vi "SendCommandTo8742.vi"(8 "error in (no error)":errorcluster, 10 "Command":string, 11 "PicoMotor8742Comm in":refnum<class "PicoMotor8742Comm.lvclass">) -> (0 "error out":errorcluster, 2 "Reply":string, 3 "PicoMotor8742Comm out":refnum<class "PicoMotor8742Comm.lvclass">)   [LabVIEW 2020, in "PicoMotor8742Comm.lvclass"]
uses:
  PicoMotor8742Comm.lvclass
  PicoMotor8742Comm.lvclass/PicoMotor8742Comm.ctl
  ASCIICommClass/ASCIICommClass.lvclass
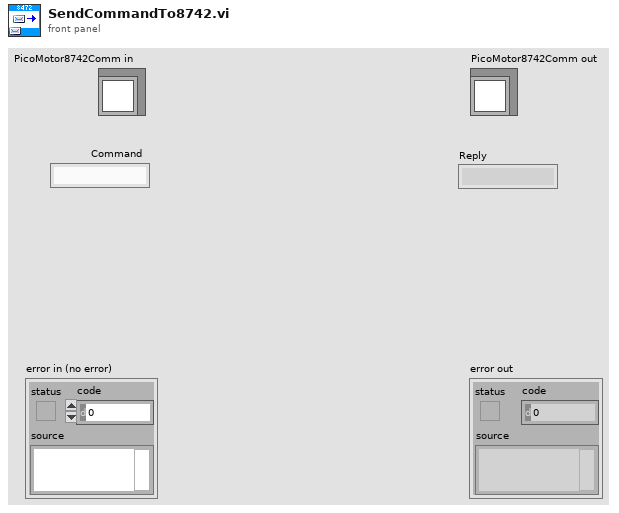
[diagram p1: front panel]
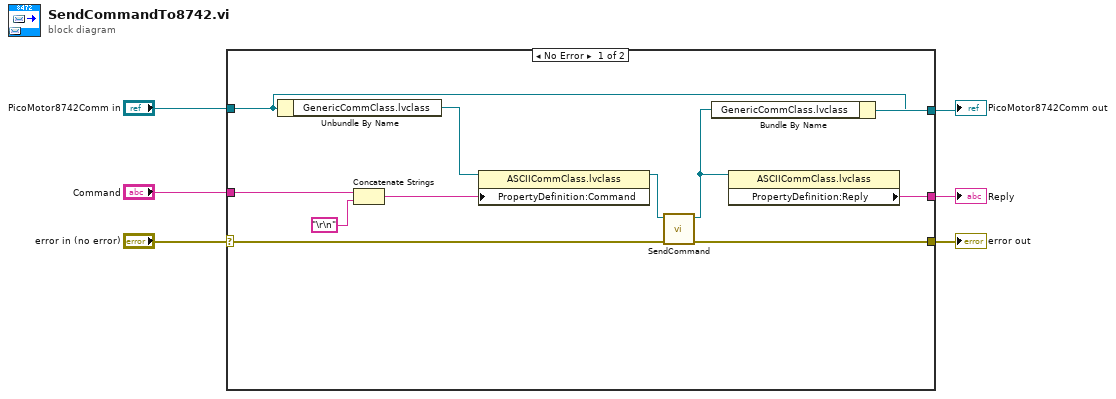
[diagram p0: block diagram]
diagram:
  n1 = case shown="No Error" "error in (no error)" {
    selector: "error in (no error)" -> [w17 w19]
    tunnel: [w16 w19] -> w5
    tunnel: "PicoMotor8742Comm in" -> [w13 w18]
    tunnel: "Command" -> [w14 _]
    tunnel: [w15 w18] -> w2
    tunnel: [w8 _] -> w1
    frame No Error {
      n2 = Unbundle By Name(w13) -> ("GenericCommClass.lvclass"=w12:refnum<class "ASCIICommClass.lvclass">)
      n3 = Concatenate Strings(w14, "\r\n") -> (w11:string)
      n4 = property class="ASCIICommClass.lvclass"(reference=w12, "PropertyDefinition:Command"=w11) -> (reference out=w10:refnum<class "ASCIICommClass.lvclass">)  [unwired: 1 in, 1 out]
      n5 = call-dynamic "SendCommand.vi"("error in (no error)"=w17, "GenericCommClass in"=w10) -> ("error out"=w16:errorcluster, "GenericCommClass out"=w9:refnum<class "ASCIICommClass.lvclass">)  [unwired: 8 in]
      n6 = Bundle By Name(cluster=w13, "GenericCommClass.lvclass"=w9) -> (w15:refnum<class "PicoMotor8742Comm.lvclass">)
      n7 = property class="ASCIICommClass.lvclass"(reference=w9) -> ("PropertyDefinition:Reply"=w8:string)  [unwired: 1 in, 2 out]
    }
    frame Error {
    }
  }
  "error out" <- w5
  "PicoMotor8742Comm out" <- w2
  "Reply" <- w1
